vi "List Columns.vi"(8 "error in (no error)":errorcluster, 10 "schema.table in":string, 11 "mysql in":refnum<class "mysql.lvclass">) -> (0 "error out":errorcluster, 2 "Columns out":string[](array[string]), 3 "mysql out":refnum<class "mysql.lvclass">, 4 "Column info out":string[][](array[string]))   [LabVIEW 2020, in "mysql.lvlib" / "mysql.lvclass"]
uses:
  mysql.lvclass
  1e5dd00d-4bc2-44a5-bcbd-962863407b88.vi
  <vilib>/Utility/error.llb/Error Cluster From Error Code.vi
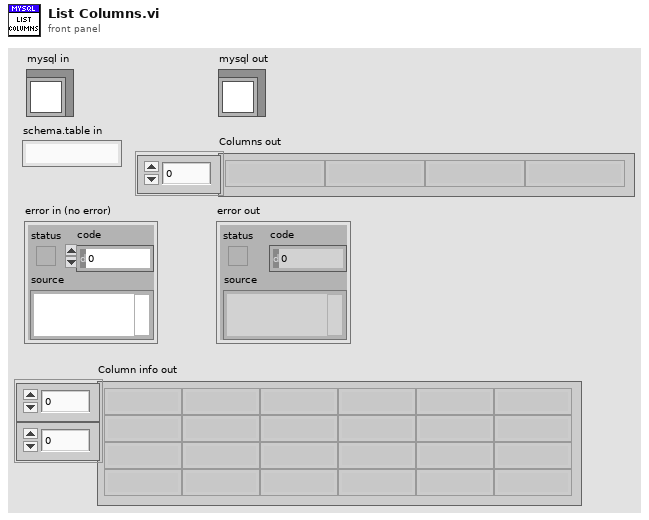
[diagram p1: front panel]
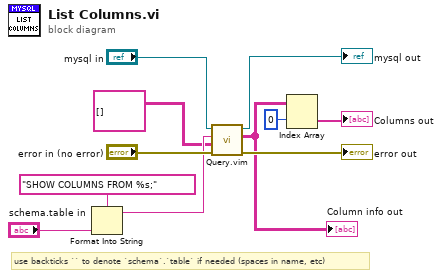
[diagram p0: block diagram]
diagram:
  # "use backticks `` to denote `schema`.`table` if needed (spaces in name, etc)"
  n1 = Format Into String(format string="SHOW COLUMNS FROM %s;" ("Query string"), "schema.table in") -> (resulting string=w6:string)  [unwired: 2 in, 1 out]
  n2 = call "Query.vim"("error in (no error)"="error in (no error)", "Type and Default"=string[][] [] ("Columns out 2"), "Query string"=w6, "IDatabase in"="mysql in") -> ("error out"=→"error out":errorcluster, "Result"=w3:string[][], "IDatabase out"=→"mysql out":refnum<class "mysql.lvclass">)  [unwired: 5 in]
  "Column info out" <- w3
  n3 = Index Array(array=w3, index (col)=0 ("disabled index (col)")) -> (element=→"Columns out":string[])  [unwired: 1 in]
